vi "HandleRightClickMenuOption.vi"(0 "reference in":refnum<class "DqmhModuleDiagramGraph.lvclass">, 1 "MenuOption":string, 2 "graphics":refnum<class "Graphics.lvclass">, 3 "grid":refnum<class "Grid.lvclass">, 4 "point":T1 {"y" format="%.2f"; "x" format="%.2f"}, 5 "error in (no error)":errorcluster) -> (14 "reference out":refnum<class "DqmhModuleDiagramGraph.lvclass">, 15 "Cancel":bool, 19 "error out":errorcluster)   [LabVIEW 2020, in "DqmhModuleDiagramGraph.lvclass"]
doc: "HandleRightClickMenuOption"
uses:
  <resource>/Framework/Providers/Open_GDS/UML/DqmhModuleDiagramGraph_class/DqmhModuleDiagramGraph.lvclass
  C:/Program Files (x86)/National Instruments/LabVIEW 2020/resource/Framework/Providers/Open_GDS/UML/Graph_class/Graph.lvclass
  <resource>/Framework/Providers/Open_GDS/UML/Graphics_class/Graphics.lvclass
  <resource>/Framework/Providers/Open_GDS/UML/Grid_class/Grid.lvclass
  <resource>/Framework/Providers/Open_GDS/UML/General/Point/Point Point2D.ctl
  <resource>/Framework/Providers/Open_GDS/UML/DQMHModuleNode_class/DQMHModuleNode.lvclass
  C:/Program Files (x86)/National Instruments/LabVIEW 2020/resource/Framework/Providers/Open_GDS/UML/AbstractNode_class/AbstractNode.lvclass
  <resource>/Framework/Providers/Open_GDS/UML/DQMHModuleNode_class/ExternalSetTypes.ctl
  <resource>/Framework/Providers/Open_GDS/UML/UMLEditor/UMLEditor_PackageClasses.ctl
  <resource>/Framework/Providers/Open_GDS/UML/AbstractNode_class/AbstractNode.lvclass
  <resource>/Framework/Providers/Open_GDS/UML/Graph_class/Graph.lvclass
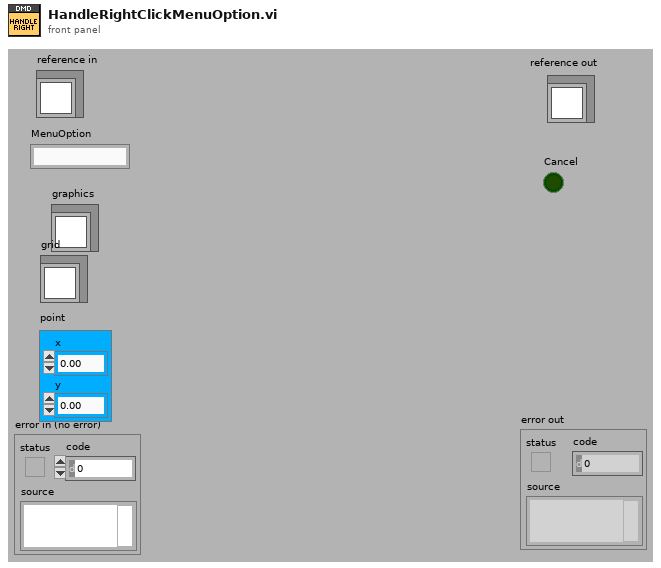
[diagram p1: front panel]
types:
  T1 = typedef "Point Point2D.ctl" = cluster{"x":dbl, "y":dbl}
  T2 = typedef "DQMHModuleNode.lvclass/ExternalSetTypes.ctl" = enum16{"Name", "Attributes", "Methods", "Position", "ShowEvents", "ShowInternalData", "ClassPath"}
  T3 = typedef "UMLEditor_PackageClasses.ctl" = cluster{"Levels":i32}
  T4 = typedef "Graph.lvclass/ObjectAttributes.ctl" = cluster{"nodes":refnum<class "AbstractNode.lvclass">[], "edges":refnum<class "AbstractEdge.lvclass">[], "nodesToBeRemoved":refnum<class "AbstractNode.lvclass">[], "edgesToBeRemoved":refnum<class "AbstractEdge.lvclass">[], "needsLayout":bool, "LayoutNodes":refnum<class "AbstractNode.lvclass">[]}
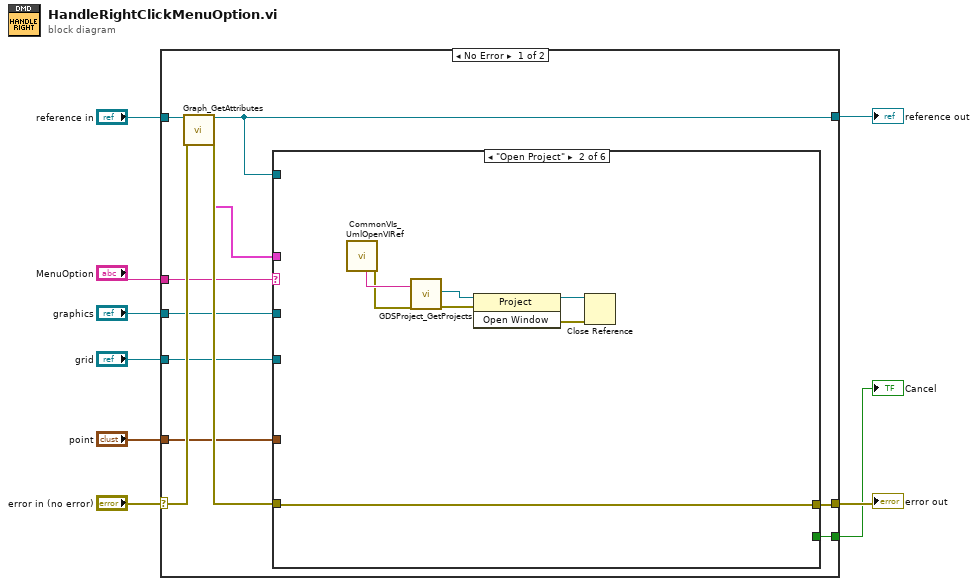
[diagram p0: block diagram]
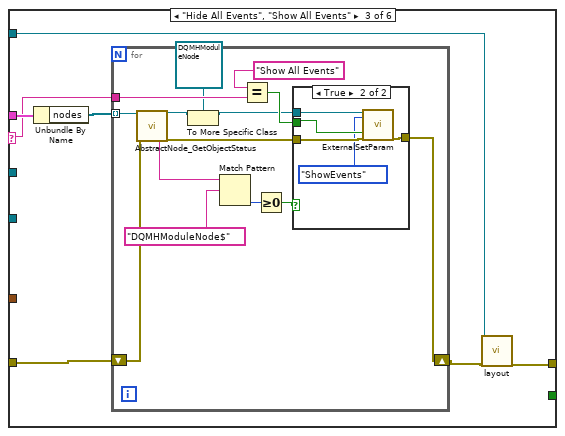
[diagram p3: hidden frame]
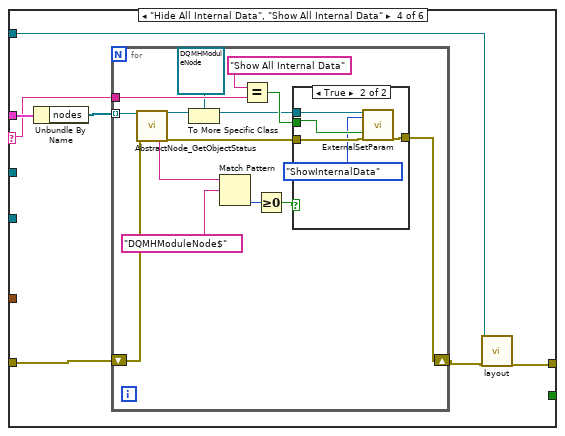
[diagram p5: hidden frame]
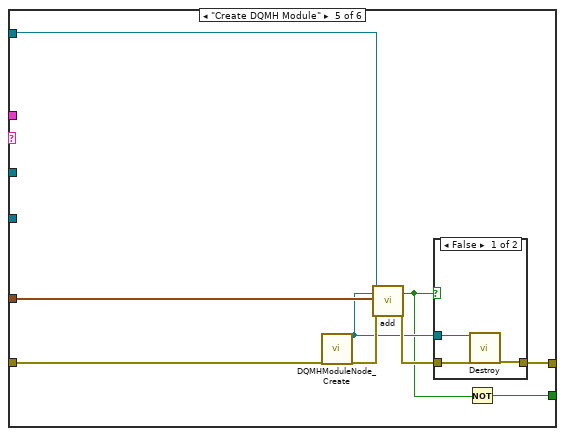
[diagram p7: hidden frame]
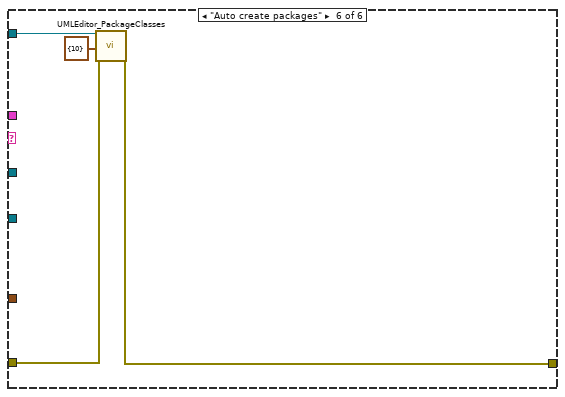
[diagram p9: hidden frame]
diagram:
  n1 = case shown="No Error" "error in (no error)" {
    selector: "error in (no error)" -> [w20 w100]
    tunnel: "reference in" -> [w19 w101]
    tunnel: [w16 w100] -> w7
    tunnel: [w17 w101] -> w6
    tunnel: "MenuOption" -> [w12 _]
    tunnel: "graphics" -> [w15 _]
    tunnel: "grid" -> [w14 _]
    tunnel: [w13 _] -> w2
    tunnel: "point" -> [w11 _]
    frame No Error {
      n2 = call <resource>:"Graph_GetAttributes.vi"("reference in"=w19, "error in (no error)"=w20) -> ("reference out"=w17:refnum<class "DqmhModuleDiagramGraph.lvclass">, "Data"=w10:T4, "error out"=w18:errorcluster)  [unwired: 14 in, 1 out]
      n3 = case shown="\"Open Project\"" w12 {
        selector: w12 -> [_ _ w32 w59 _ _]
        tunnel: w18 -> [w21 w22 w34 w61 w88 w98]
        tunnel: w17 -> [_ _ w29 w56 w87 w99]
        tunnel: [w21 w22 w30 w57 w90 w97] -> w16
        tunnel: w10 -> [_ _ w35 w62 _ _]
        tunnel: w15 -> [_ _ _ _ _ _]
        tunnel: w14 -> [_ _ _ _ _ _]
        tunnel: [_ _ _ _ w89 _] -> w13
        tunnel: w11 -> [_ _ _ _ w91 _]
        frame "False", Default {
        }
        frame "Open Project" {
          n4 = call <resource>:"CommonVIs_UmlOpenVIRef.vi"() -> ("error out"=w27:errorcluster, "ProjectNameOut"=w28:string)  [unwired: 4 in, 6 out]
          n5 = call <resource>:"GDSProject_GetProjects.vi"("GetProjectRefByName"=w28, "error in (no error)"=w27) -> ("Project Refnum"=w26:refnum<vi>, "error out"=w25:errorcluster)  [unwired: 1 in, 15 out]
          n6 = invoke class="Project" method="Open Window"(reference=w26, error in=w25) -> (reference out=w23:refnum<vi>, error out=w24:errorcluster)  [unwired: 1 in, 1 out]
          n7 = Close Reference(reference=w23, error in (no error)=w24) -> ()  [unwired: 1 out]
        }
        frame "Hide All Events", "Show All Events" {
          n8 = Unbundle By Name(w35) -> ("nodes"=w33:refnum<class "AbstractNode.lvclass">[])
          n9 = for {
            shift-right: [w40] -> w31
            shift-left: w34 -> [w48]
            tunnel: w33 -> [w49] mode=indexing
            tunnel: w32 -> [w44]
            n10 = call <resource>:"AbstractNode_GetObjectStatus.vi"("reference in"=w49, "error in (no error)"=w48) -> ("Class name"=w36:string, "reference out"=w39:refnum<class "AbstractNode.lvclass">, "error out"=w41:errorcluster)  [unwired: 15 out]
            n11 = To More Specific Class(target class=refnum<class "DQMHModuleNode.lvclass"> refnum ("reference"), reference=w39) -> (specific class reference=w38:refnum<class "DQMHModuleNode.lvclass">)  [unwired: 1 in, 1 out]
            n12 = Match Pattern(string=w36, regular expression="DQMHModuleNode$") -> (offset past match=w46:i32)  [unwired: 4 out]
            n13 = Equal?(x="Show All Events", y=w44) -> (x = y?=w42:bool)
            n14 = Greater Or Equal To 0?(x=w46) -> (x >= 0?=w45:bool)
            n15 = case shown="True" w45 {
              tunnel: w42 -> [_ w52]
              tunnel: w38 -> [_ w55]
              tunnel: w41 -> [w50 w54]
              tunnel: [w50 w53] -> w40
              frame False {
              }
              frame True {
                n16 = call-dynamic "ExternalSetParam.vi"("reference in"=w55, "setParameter"=ExternalSetTypes."ShowEvents", "Boolean"=w52, "error in (no error)"=w54) -> ("error out"=w53:errorcluster)  [unwired: 14 in, 1 out]
              }
            }
          }
          n17 = call-dynamic "layout.vi"("reference"=w29, "error in (no error)"=w31) -> ("error out"=w30:errorcluster)  [unwired: 16 in, 1 out]
        }
        frame "Hide All Internal Data", "Show All Internal Data" {
          n18 = Unbundle By Name(w62) -> ("nodes"=w60:refnum<class "AbstractNode.lvclass">[])
          n19 = for {
            shift-right: [w67] -> w58
            shift-left: w61 -> [w75]
            tunnel: w60 -> [w76] mode=indexing
            tunnel: w59 -> [w71]
            n20 = call <resource>:"AbstractNode_GetObjectStatus.vi"("reference in"=w76, "error in (no error)"=w75) -> ("Class name"=w64:string, "reference out"=w66:refnum<class "AbstractNode.lvclass">, "error out"=w68:errorcluster)  [unwired: 15 out]
            n21 = To More Specific Class(target class=refnum<class "DQMHModuleNode.lvclass"> refnum ("reference"), reference=w66) -> (specific class reference=w65:refnum<class "DQMHModuleNode.lvclass">)  [unwired: 1 in, 1 out]
            n22 = Match Pattern(string=w64, regular expression="DQMHModuleNode$") -> (offset past match=w73:i32)  [unwired: 4 out]
            n23 = Equal?(x="Show All Internal Data", y=w71) -> (x = y?=w69:bool)
            n24 = Greater Or Equal To 0?(x=w73) -> (x >= 0?=w72:bool)
            n25 = case shown="True" w72 {
              tunnel: w69 -> [_ w79]
              tunnel: w65 -> [_ w82]
              tunnel: w68 -> [w77 w81]
              tunnel: [w77 w80] -> w67
              frame False {
              }
              frame True {
                n26 = call-dynamic "ExternalSetParam.vi"("reference in"=w82, "setParameter"=ExternalSetTypes."ShowInternalData", "Boolean"=w79, "error in (no error)"=w81) -> ("error out"=w80:errorcluster)  [unwired: 14 in, 1 out]
              }
            }
          }
          n27 = call-dynamic "layout.vi"("reference"=w56, "error in (no error)"=w58) -> ("error out"=w57:errorcluster)  [unwired: 16 in, 1 out]
        }
        frame "Create DQMH Module" {
          n28 = call <resource>:"DQMHModuleNode_Create.vi"("error in (no error)"=w88) -> ("reference out"=w84:refnum<class "DQMHModuleNode.lvclass">, "error out"=w86:errorcluster)  [unwired: 17 in]
          n29 = call-dynamic "add.vi"("reference"=w87, "node"=w84, "point"=w91, "error in (no error)"=w86) -> ("added"=w83:bool, "error out"=w85:errorcluster)  [unwired: 13 in, 1 out]
          n30 = case shown="False" w83 {
            tunnel: w85 -> [w94 w95]
            tunnel: [w93 w95] -> w90
            tunnel: w84 -> [w92 _]
            frame False {
              n31 = call-dynamic "Destroy.vi"("reference in"=w92, "error in (no error)"=w94) -> ("error out"=w93:errorcluster)  [unwired: 16 in, 1 out]
            }
            frame True {
            }
          }
          n32 = Not(x=w83) -> (.not. x?=w89:bool)
        }
        frame "Auto create packages" {
          n33 = call <resource>:"UMLEditor_PackageClasses.vi"("DiagramIn"=w99, "Settings"=T3 {"Levels"=10}, "error in (no error)"=w98) -> ("error out"=w97:errorcluster)  [unwired: 16 in]
        }
      }
    }
    frame Error {
    }
  }
  "reference out" <- w6
  "error out" <- w7
  "Cancel" <- w2
